vi "Read_Modbus_VI.vi"(8 "error in (no error)":errorcluster, 10 "millisecond timer value":u32, 11 "Modbus master in":refnum<class "Modbus Master.lvclass">) -> (0 "error out":errorcluster, 1 "Execution Rate":dbl, 2 "All Parameters":u16[](array[numeric]), 3 "Modbus master out":refnum<class "Modbus Master.lvclass">)   [LabVIEW 2021]
uses:
  <vilib>/Modbus/master/Modbus Master.lvclass
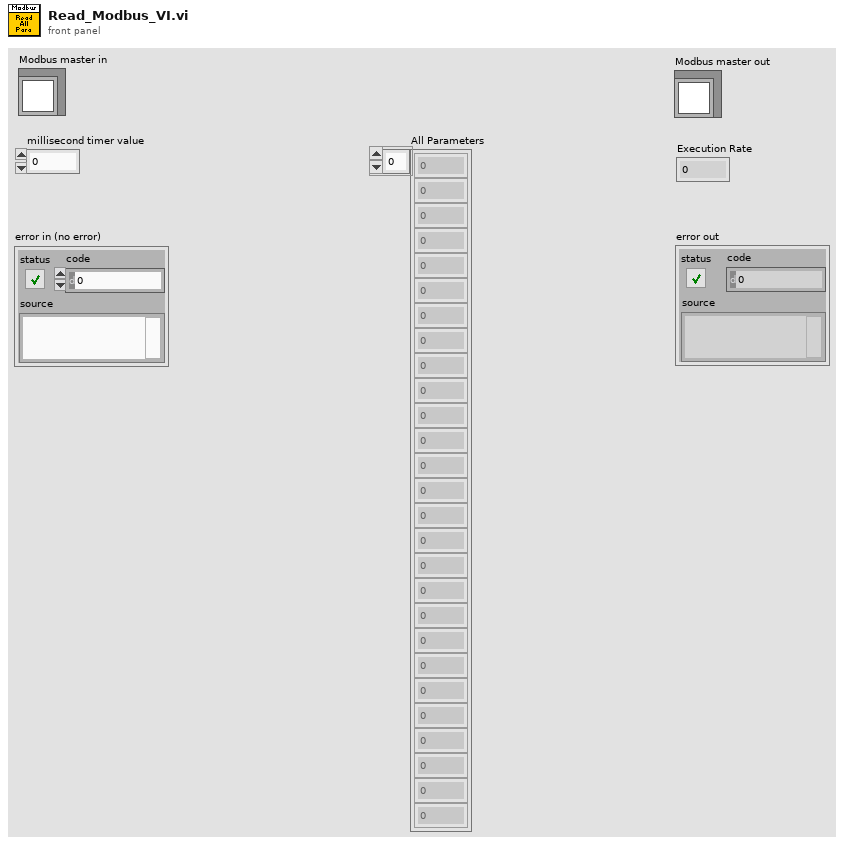
[diagram p1: front panel]
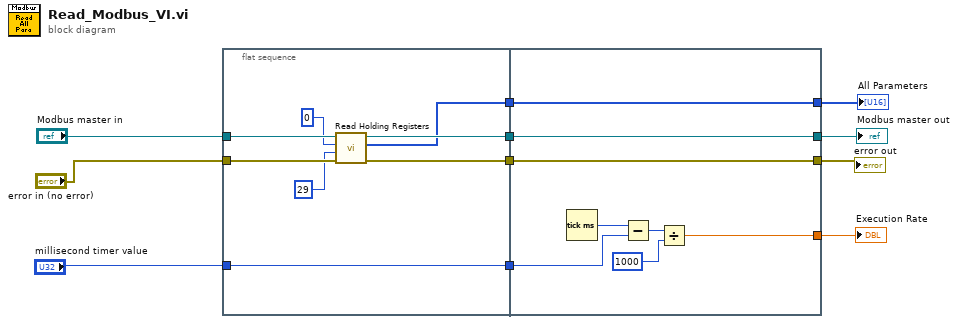
[diagram p0: block diagram]
diagram:
  n1 = flat-sequence {
    tunnel: "Modbus master in" -> [w19]
    tunnel: "error in (no error)" -> [w18]
    tunnel: [w17] -> w7
    tunnel: [w16] -> w6
    tunnel: [w13] -> w4
    tunnel: "millisecond timer value" -> [w13]
    tunnel: [w12] -> w2
    tunnel: [w26] -> w8
    tunnel: [w27] -> w9
    tunnel: w7 -> [w27]
    tunnel: w6 -> [w26]
    tunnel: [w22] -> w5
    tunnel: w4 -> [w21]
    tunnel: [w20] -> w1
    tunnel: w2 -> [w20]
    frame #0 {
      n2 = call-dynamic "Read Holding Registers.vi"("error in (no error)"=w18, "number of holding registers"=u16 29, "starting address"=u16 0, "Modbus master in"=w19) -> ("error out"=w16:errorcluster, "register values"=w12:u16[], "Modbus master out"=w17:refnum<class "Modbus Master.lvclass">)  [unwired: 5 in]
    }
    frame #1 {
      n3 = Tick Count (ms)() -> (millisecond timer value=w24:u32)
      n4 = Subtract(x=w24, y=w21) -> (x-y=w25:u32)
      n5 = Divide(x=w25, y=u32 1000) -> (x/y=w22:dbl)
    }
  }
  "Modbus master out" <- w9
  "error out" <- w8
  "Execution Rate" <- w5
  "All Parameters" <- w1
